vi "auto_mode.vi"(4 "Curve":i8, 5 "Base Position":bool, 6 "Back":bool, 7 "POWER":bool, 8 "Right":bool, 9 "Forth":bool, 10 "Left":bool, 11 "Speed":u8(slide)=1 scale=1.0..10.0) -> (3 "String":string)   [LabVIEW 2012]
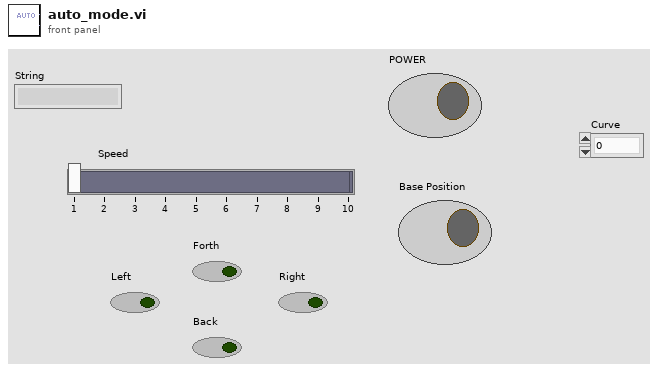
[diagram p1: front panel]
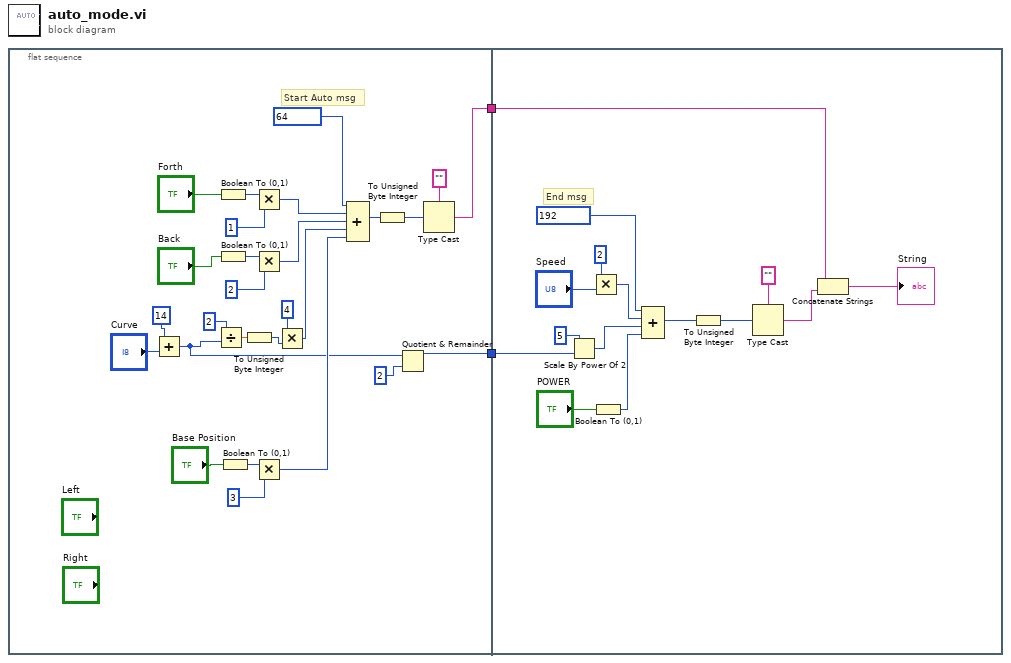
[diagram p0: block diagram]
diagram:
  n1 = flat-sequence {
    tunnel: [w23] -> w2
    tunnel: [w7] -> w1
    tunnel: w2 -> [w43]
    tunnel: w1 -> [w30]
    frame #0 {
      # "Start Auto msg"
      n2 = Add(x=i8 14, y="Curve") -> (x+y=w6:i8)
      n3 = Divide(x=w6, y=i8 2) -> (x/y=w3:dbl)
      n4 = Boolean To (0,1)(Boolean="Forth") -> (0, 1=w28:i16)
      n5 = Boolean To (0,1)(Boolean="Back") -> (0, 1=w22:i16)
      n6 = Boolean To (0,1)(Boolean="Base Position") -> (0, 1=w16:i16)
      n7 = To Unsigned Byte Integer(number=w3) -> (unsigned 8bit integer=w4:u8)
      n8 = Multiply(x=w28, y=i16 1) -> (x*y=w19:i16)
      n9 = Multiply(x=w22, y=i16 2) -> (x*y=w18:i16)
      n10 = Multiply(x=w16, y=i16 3) -> (x*y=w10:i16)
      n11 = Multiply(x=i8 4, y=w4) -> (x*y=w9:u8)
      n12 = Compound Arithmetic op=ADD(u8 64, w19, w18, w9, w10) -> (w25:i16)
      n13 = To Unsigned Byte Integer(number=w25) -> (unsigned 8bit integer=w24:u8)
      n14 = Quotient & Remainder(x=w6, y=i16 2) -> (x-y*floor(x/y)=w7:i16)  [unwired: 1 out]
      n15 = Type Cast(type="", x=w24) -> (*(type *) &x=w23:string)
    }
    frame #1 {
      # "End msg"
      n16 = Scale By Power Of 2(n=i16 5, x=w30) -> (x*2^n=w31:i16)
      n17 = Multiply(x=u8 2, y="Speed") -> (x*y=w40:u8)
      n18 = Boolean To (0,1)(Boolean="POWER") -> (0, 1=w32:i16)
      n19 = Compound Arithmetic op=unknown(192, w40, w31, w32) -> (w35:i32)
      n20 = To Unsigned Byte Integer(number=w35) -> (unsigned 8bit integer=w34:u8)
      n21 = Type Cast(type="", x=w34) -> (*(type *) &x=w36:string)
      n22 = Concatenate Strings(w43, w36) -> (→"String":string)
    }
  }
